vi "DFD Dolph-Chebyshev Order Estimation.vi"(6 "fs [Hz]":dbl=1.0 format="%.2f", 7 "filter type":T3(ring), 8 "error in (no error)":errorcluster, 9 "order option":enum16{"MinNum", "MinEven", "MinOdd"}(ring)=enum."MinEven", 10 "ripple specs":T1={"passband"=0.1, "stopband"=60.0, "dB/linear? (T: dB)"=TRUE}, 11 "freq specs [Hz]":T2={"fpass 1"=0.2, "fstop 1"=0.3, "fpass 2 "=0.0, "fstop 2"=0.0}) -> (0 "error out":errorcluster, 1 "low cutoff freq [Hz]":dbl, 2 "high cutoff freq [Hz]":dbl, 3 "estimated order":i32, 4 "ripple ratio [dB]":dbl format="%.2f")   [LabVIEW 2017, in "NI_DigFilterLicensed.lvlib"]
doc: "Estimates the order of a finite impulse response (FIR) filter that you designed by using the Dolph-Chebyshev Window method."
uses:
  <vilib>/addons/Digital Filter Design/NI_DigFilterLicensed.lvlib
  <vilib>/addons/Digital Filter Design/_Objects.llb/DFD Filter Frequence Specification (Design).ctl
  <vilib>/addons/Digital Filter Design/_Objects.llb/DFD Filter Ripple Specification (Design).ctl
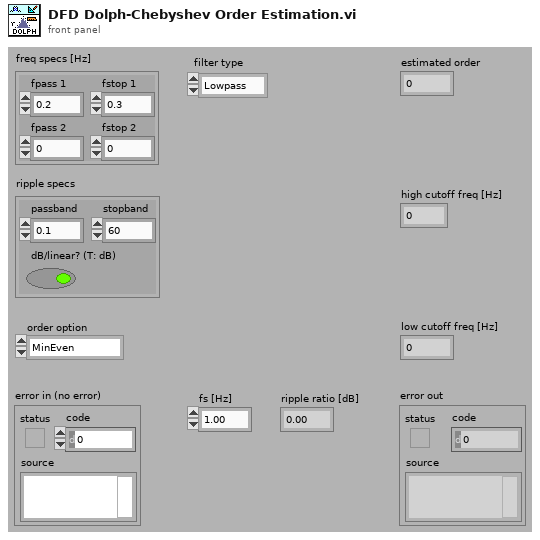
[diagram p1: front panel]
types:
  T1 = typedef "NI_DigFilterLicensed.lvlib/DFD Filter Ripple Specification (Design).ctl" = cluster{"passband":dbl, "stopband":dbl, "dB/linear? (T: dB)":bool}
  T2 = typedef "NI_DigFilterLicensed.lvlib/DFD Filter Frequence Specification (Design).ctl" = cluster{"fpass 1":dbl, "fstop 1":dbl, "fpass 2 ":dbl, "fstop 2":dbl}
  T3 = enum16{"Lowpass", "Highpass", "Bandpass", "Bandstop"}
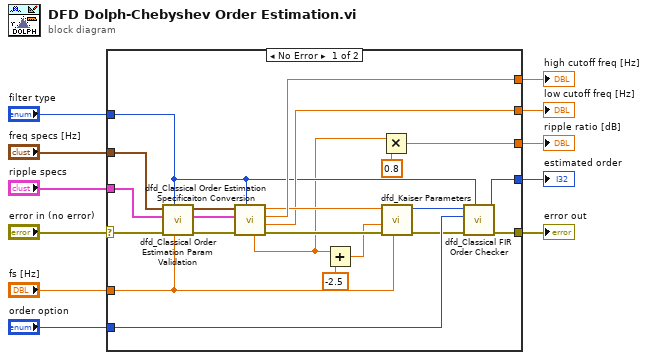
[diagram p0: block diagram]
diagram:
  n1 = case shown="No Error" "error in (no error)" {
    selector: "error in (no error)" -> [w12 w34]
    tunnel: [w33 _] -> w11
    tunnel: [w32 w34] -> w10
    tunnel: "order option" -> [w31 _]
    tunnel: "fs [Hz]" -> [w29 _]
    tunnel: "freq specs [Hz]" -> [w23 _]
    tunnel: "ripple specs" -> [w21 _]
    tunnel: [w19 _] -> w5
    tunnel: [w16 _] -> w4
    tunnel: "filter type" -> [w15 _]
    tunnel: [w13 _] -> w2
    frame No Error {
      n2 = call <vilib>:"dfd_Classical Order Estimation Param Validation.vi"("fs [Hz]"=w29, "filter type"=w15, "error in (no error)"=w12, "ripple specs"=w21, "freq specs [Hz]"=w23) -> ("error out"=w30:errorcluster, "dup ripple specs"=w20:T1, "dup freq specs [Hz]"=w22:T2)  [unwired: 1 in, 3 out]
      n3 = call <vilib>:"dfd_Classical Order Estimation Specificaiton Conversion.vi"("filter type"=w15, "error in (no error)"=w30, "ripple specs"=w20, "freq specs [Hz]"=w22) -> ("error out"=w24:errorcluster, "low cutoff freq: fl"=w19:dbl, "high cutoff freq: fh"=w33:dbl, "min transition band"=w28:dbl, "A stop (dB)"=w14:dbl)  [unwired: 1 in, 2 out]
      n4 = Add(x=w14, y=-2.5) -> (x+y=w18:dbl)
      n5 = Multiply(x=w14, y=0.8) -> (x*y=w16:dbl)
      n6 = call <vilib>:"dfd_Kaiser Parameters.vi"("fs [Hz]"=w29, "error in (no error)"=w24, "A stop [dB]"=w18, "delta f [Hz]"=w28) -> ("error out"=w25:errorcluster, "order"=w27:i32)  [unwired: 1 in, 5 out]
      n7 = call <vilib>:"dfd_Classical FIR Order Checker.vi"("filter type"=w15, "error in (no error)"=w25, "order option"=w31, "order in"=w27) -> ("error out"=w32:errorcluster, "order out"=w13:i32)  [unwired: 6 out]
    }
    frame Error {
    }
  }
  "error out" <- w10
  "estimated order" <- w2
  "ripple ratio [dB]" <- w4
  "high cutoff freq [Hz]" <- w11
  "low cutoff freq [Hz]" <- w5
